vi "Acquire.vi"(8 "error in (no error)":errorcluster, 9 "queue out":refnum<queue>, 10 "notifier out":refnum<notifier>, 11 "Hardware Resources in":T1) -> (0 "error out":errorcluster, 3 "Hardware Resources out":T1)   [LabVIEW 2019, in "Acquisition.lvlib"]
doc: "Perform the acquisition. Replace the contents of this diagram with calls to acquisition hardware."
uses:
  Acquisition.lvlib
  Hardware Configuration.ctl
  <vilib>/DAQmx/read.llb/DAQmx Read (Analog 1D Wfm NChan NSamp).vi
  <vilib>/DAQmx/write.llb/DAQmx Write (Analog 1D DBL NChan 1Samp).vi
  Global Thermistor Coefficient Array.vi
  Settings/Global Excitation Current.vi
  <vilib>/DAQmx/miscellaneous.llb/DAQmx Fill In Error Info.vi
  <resource>/objmgr/daqmx.rc
  Analysis/Analysis.lvlib
panel:
  out "Waveform Graph":waveform(dbl)[](graph)
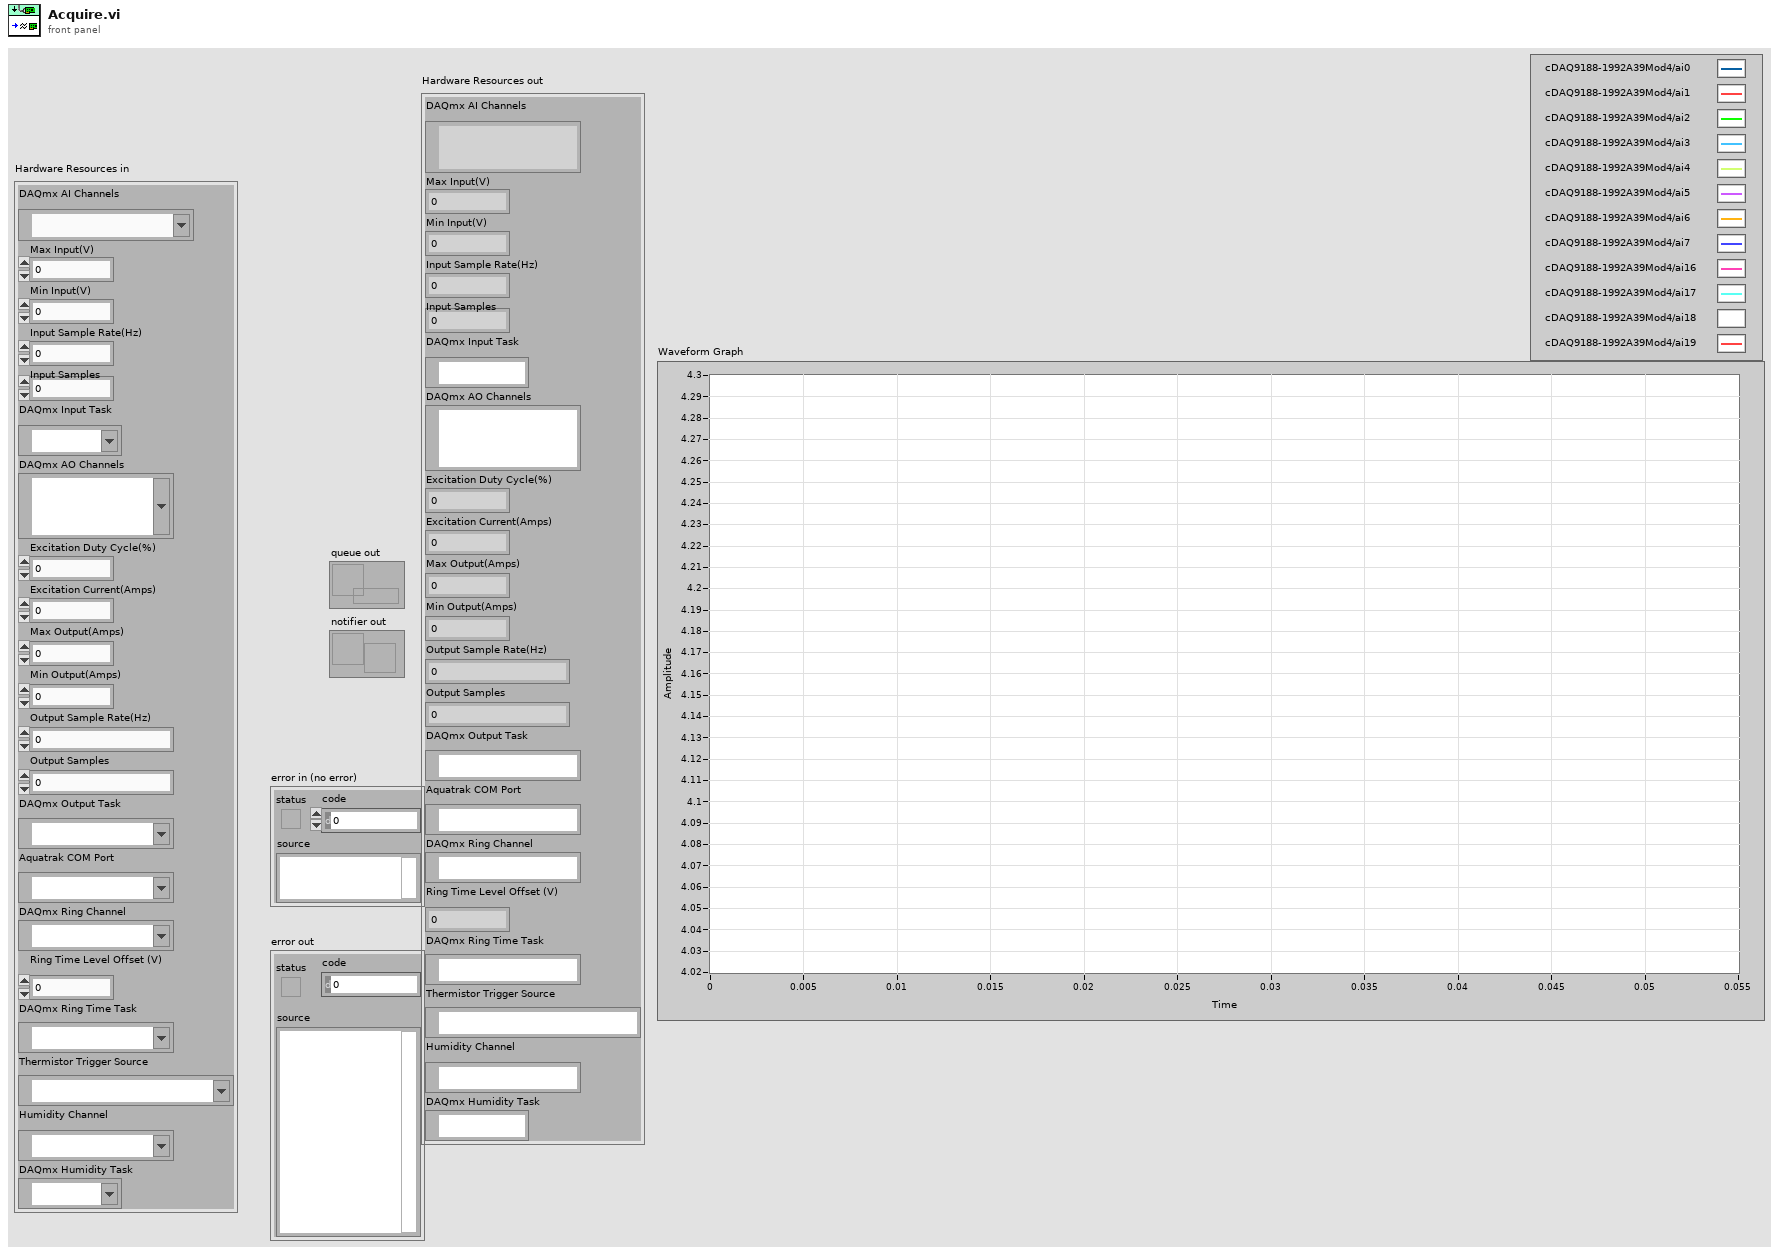
[diagram p1: front panel]
types:
  T1 = typedef "Acquisition.lvlib/Hardware Configuration.ctl" = cluster{"DAQmx AI Channels":tag, "Max Input(V)":dbl, "Min Input(V)":dbl, "Input Sample Rate(Hz)":dbl, "Input Samples":dbl, "DAQmx Input Task":refnum<k21>, "DAQmx AO Channels":tag, "Excitation Duty Cycle(%)":dbl, "Excitation Current(Amps)":dbl, "Max Output(Amps)":dbl, "Min Output(Amps)":dbl, "Output Sample Rate(Hz)":dbl, "Output Samples":dbl, "DAQmx Output Task":refnum<k21>, "Aquatrak COM Port":refnum<visa-resource-name>, "DAQmx Ring Channel":tag, "Ring Time Level Offset (V)":dbl, "DAQmx Ring Time Task":refnum<k21>, "Thermistor Trigger Source":tag, "Humidity Channel":tag, "DAQmx Humidity Task":refnum<k21>}
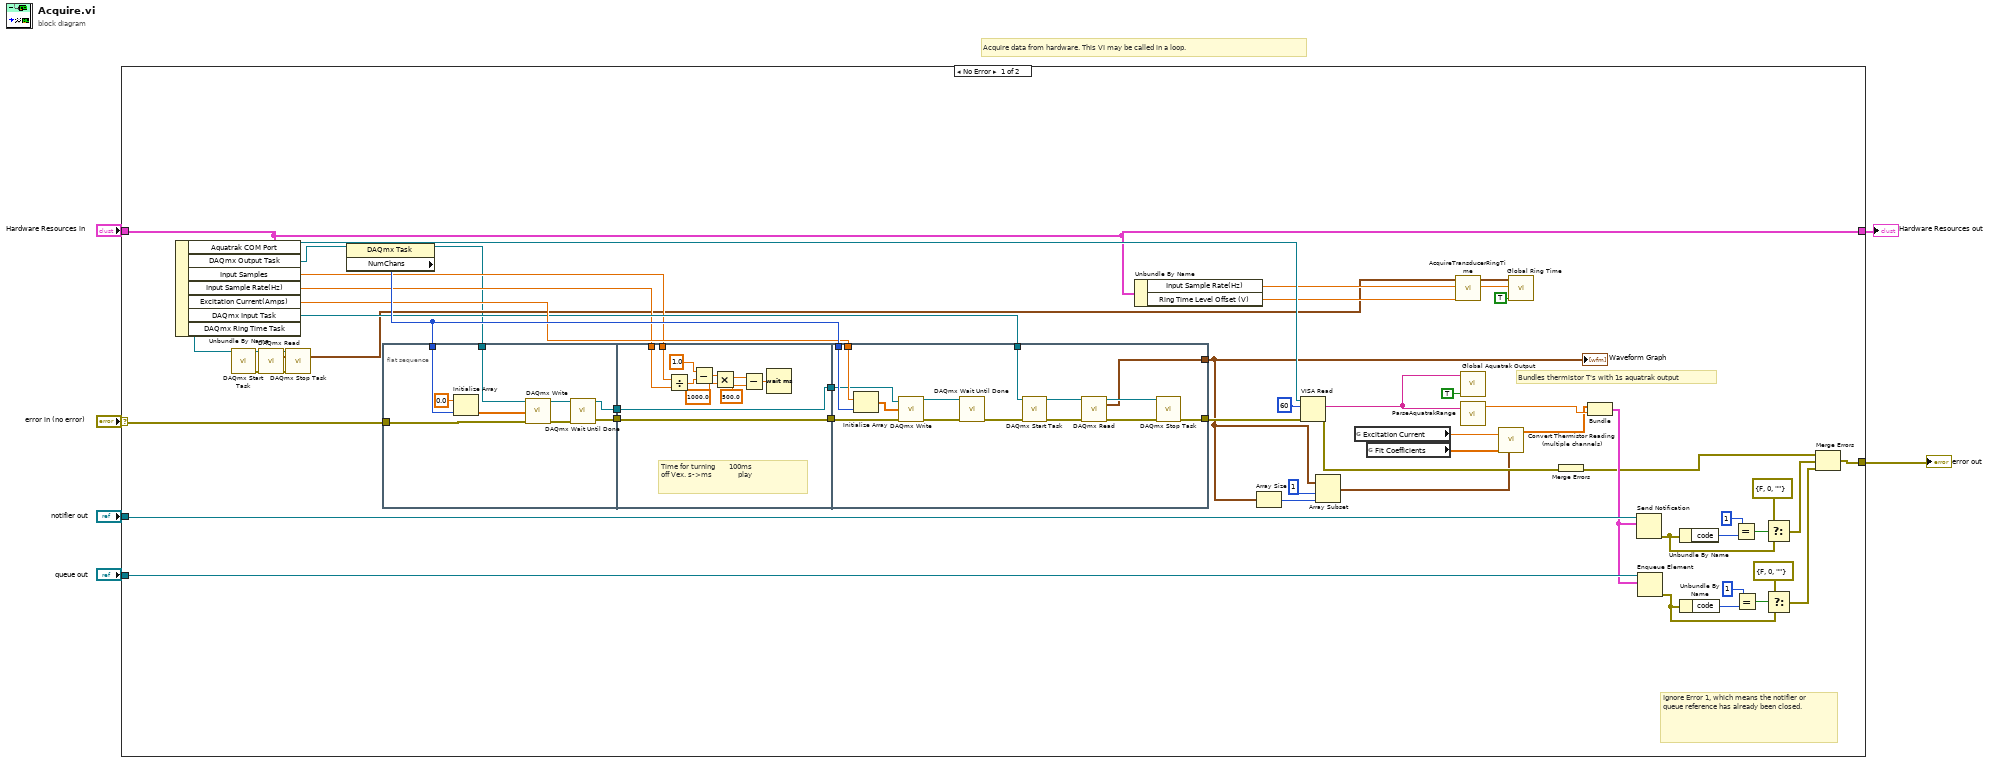
[diagram p0: block diagram]
diagram:
  # "Acquire data from hardware. This VI may be called in a loop."
  n1 = case shown="No Error" "error in (no error)" {
    selector: "error in (no error)" -> [w22 w97]
    tunnel: [w61 w97] -> w5
    tunnel: "Hardware Resources in" -> [w30 w98]
    tunnel: [w30 w98] -> w3
    tunnel: "notifier out" -> [w60 _]
    tunnel: "queue out" -> [w47 _]
    frame No Error {
      # "Bundles thermistor T's with 1s aquatrak output"
      # "Ignore Error 1, which means the notifier or queue reference has already been closed."
      n2 = Unbundle By Name(w30) -> ("Aquatrak COM Port"=w43:refnum<visa-resource-name>, "DAQmx Output Task"=w8:refnum<k21>, "Input Samples"=w37:dbl, "Input Sample Rate(Hz)"=w36:dbl, "Excitation Current(Amps)"=w40:dbl, "DAQmx Input Task"=w39:refnum<k21>, "DAQmx Ring Time Task"=w23:refnum<k21>)
      n3 = call <vilib>:"DAQmx Start Task.vi"("task/channels in"=w23) -> ("task out"=w27:refnum<k21>, "error out"=w26:errorcluster)  [unwired: 13 in]
      n4 = call-poly <vilib>:"DAQmx Read.vi"("task/channels in"=w27, "error in"=w26) -> ("task out"=w24:refnum<k21>, "data"=w21:waveform(dbl)[], "error out"=w25:errorcluster)  [unwired: 11 in]
      n5 = call <vilib>:"DAQmx Stop Task.vi"("task/channels in"=w24, "error in"=w25) -> ()  [unwired: 12 in, 2 out]
      n6 = property class="DAQmx Task"(reference=w8) -> (reference out=w7:refnum<k21>, "NumChans"=w45:u32)  [unwired: 1 in, 1 out]
      n7 = flat-sequence {
        tunnel: w45 -> [w69]
        tunnel: w7 -> [w70]
        tunnel: [w64] -> w38
        tunnel: w22 -> [w63]
        tunnel: [w62] -> w9
        tunnel: [w81] -> w41
        tunnel: w38 -> [w81]
        tunnel: w36 -> [w73]
        tunnel: w37 -> [w72]
        tunnel: [w71] -> w10
        tunnel: w9 -> [w71]
        tunnel: [w87] -> w42
        tunnel: w40 -> [w94]
        tunnel: w45 -> [w83]
        tunnel: w41 -> [w95]
        tunnel: w39 -> [w85]
        tunnel: [w84] -> w18
        tunnel: w10 -> [w82]
        frame #0 {
          n8 = Initialize Array(0.0 ("element"), w69) -> (w68:dbl[])
          n9 = call-poly <vilib>:"DAQmx Write.vi"("task/channels in"=w70, "data"=w68, "error in"=w63) -> ("task out"=w66:refnum<k21>, "error out"=w67:errorcluster)  [unwired: 10 in, 1 out]
          n10 = call <vilib>:"DAQmx Wait Until Done.vi"("task/channels in"=w66, "error in"=w67) -> ("task out"=w62:refnum<k21>, "error out"=w64:errorcluster)  [unwired: 12 in]
        }
        frame #1 {
          # "Time for turning       100ms\noff Vex. s->ms             play"
          n11 = Divide(x=w72, y=w73) -> (x/y=w75:dbl)
          n12 = Subtract(x=1.0, y=w75) -> (x-y=w77:dbl)
          n13 = Multiply(x=w77, y=1000.0 ("x")) -> (x*y=w80:dbl)
          n14 = Subtract(x=w80, y=500.0 ("x")) -> (x-y=w78:dbl)
          n15 = Wait (ms)(milliseconds to wait=w78) -> ()  [unwired: 1 out]
        }
        frame #2 {
          n16 = Initialize Array(w94, w83) -> (w96:dbl[])
          n17 = call-poly <vilib>:"DAQmx Write.vi"("task/channels in"=w82, "data"=w96, "error in"=w95) -> ("task out"=w92:refnum<k21>, "error out"=w93:errorcluster)  [unwired: 10 in, 1 out]
          n18 = call <vilib>:"DAQmx Wait Until Done.vi"("task/channels in"=w92, "error in"=w93) -> ("error out"=w86:errorcluster)  [unwired: 12 in, 1 out]
          n19 = call <vilib>:"DAQmx Start Task.vi"("task/channels in"=w85, "error in"=w86) -> ("task out"=w88:refnum<k21>, "error out"=w89:errorcluster)  [unwired: 12 in]
          n20 = call-poly <vilib>:"DAQmx Read.vi"("task/channels in"=w88, "error in"=w89) -> ("task out"=w91:refnum<k21>, "data"=w84:waveform(dbl)[], "error out"=w90:errorcluster)  [unwired: 11 in]
          n21 = call <vilib>:"DAQmx Stop Task.vi"("task/channels in"=w91, "error in"=w90) -> ("error out"=w87:errorcluster)  [unwired: 12 in, 1 out]
        }
      }
      n22 = Unbundle By Name(w30) -> ("Input Sample Rate(Hz)"=w28:dbl, "Ring Time Level Offset (V)"=w29:dbl)
      n23 = Array Size(array=w18) -> (size(s)=w20:i32)
      n24 = VISA Read(VISA resource name=w43, byte count=u32 60, error in (no error)=w42) -> (read buffer=w12:string, error out=w34:errorcluster)  [unwired: 2 out]
      n25 = Array Subset(array=w18, index=1 ("size(s)"), length=w20) -> (w15:waveform(dbl)[])
      n26 = global read "Global Excitation Current.vi" "Excitation Current"() -> (w17:dbl)
      n27 = global read "Global Thermistor Coefficient Array.vi" "Fit Coefficients"() -> (w16:dbl[][])
      n28 = call "AcquireTransducerRingTime.vi"("Cut-Off Level"=w29, "Sampling Rate"=w28, "Ring Time Wavefrom Array"=w21) -> ("Ring Time (ms)"=w31:dbl, "Measurement"=w32:waveform(dbl))  [unwired: 6 in, 1 out]
      n29 = call "Global Aquatrak Output.vi"("AT In"=w12, "Set Data?"=TRUE) -> ()  [unwired: 8 in, 1 out]
      n30 = call "ParseAquatrakRange.vi"("Incoming String"=w12) -> ("Range"=w14:dbl)  [unwired: 6 in, 4 out]
      n31 = call "Convert Thermistor Reading (multiple channels).vi"("Voltage Array"=w15, "Fit Coefficients"=w16, "Excitation Current"=w17) -> ("Temperature Array"=w13:dbl[])  [unwired: 7 in, 1 out]
      n32 = call "Global Ring Time.vi"("Ring Time Plot In"=w32, "Ring Time (ms) In"=w31, "Set Data?"=TRUE) -> ()  [unwired: 6 in, 2 out]
      n33 = Merge Errors(w34) -> (w35:errorcluster)
      n34 = Bundle("Temperature Array"=w13, "Range"=w14) -> (w46:cluster{"Temperature Array":dbl[], "Range":dbl})  [unwired: 1 in]
      n35 = Send Notification(notification=w46, notifier=w60) -> (error out=w56:errorcluster)  [unwired: 1 in, 1 out]
      n36 = Enqueue Element(queue=w47, element=w46) -> (error out=w52:errorcluster)  [unwired: 2 in, 2 out]
      n37 = Unbundle By Name(w56) -> ("code"=w59:i32)
      n38 = Unbundle By Name(w52) -> ("code"=w49:i32)
      n39 = Equal?(x=1, y=w59) -> (x = y?=w57:bool)
      n40 = Equal?(x=1, y=w49) -> (x = y?=w51:bool)
      n41 = Select(t=errorcluster {"status"=FALSE, "code"=0, "source"=""} ("error constant"), s=w57, f=w56) -> (s? t:f=w55:errorcluster)
      n42 = Select(t=errorcluster {"status"=FALSE, "code"=0, "source"=""} ("error constant"), s=w51, f=w52) -> (s? t:f=w48:errorcluster)
      n43 = Merge Errors(w35, w55, w48) -> (w61:errorcluster)
      "Waveform Graph" <- w18
    }
    frame Error {
    }
  }
  "Hardware Resources out" <- w3
  "error out" <- w5
